vi "Send Initialize Range Controller.vi"(6 "Main Controls":refnum<vi>, 7 "Priority":T3=enum."Normal" caption="Message Priority (Normal)", 8 "error in (no error)":errorcluster, 9 "Ranges Refnum":T1, 10 "Settings":T2, 11 "Message Enqueuer in":refnum<class "Message Enqueuer.lvclass">) -> (0 "error out":errorcluster, 3 "Message Enqueuer out":refnum<class "Message Enqueuer.lvclass">)   [LabVIEW 2018, in "Range Controller.lvlib" / "Initialize Range Controller Msg.lvclass"]
doc: "Sends the <b>Range Controller.lvlib:Initialize Range Controller Msg.lvclass</b> message.\n\nThis message will call <b>Initialize Range Controller.vi</b> on the <b>Range Controller.lvlib:Range Controller Actor.lvclass</b> actor.\n\n<b>Initialize Range Controller.vi Description</b>"
uses:
  Initialize Range Controller Msg.lvclass
  <vilib>/ActorFramework/Message Enqueuer/Message Enqueuer.lvclass
  <vilib>/ActorFramework/Message Enqueuer/Message Priority.ctl
  MWWL Verification/Type Defs/ConfigSettings.ctl
  MWWL Verification/MWWL Verification/Ranges Refnum.ctl
  C:/Program Files (x86)/National Instruments/LabVIEW 2018/vi.lib/ActorFramework/Message/Message.lvclass
  Initialize Range Controller Msg.lvclass/Initialize Range Controller Msg.ctl
  <vilib>/ActorFramework/Message Enqueuer/Message Enqueuer.lvclass/Message Enqueuer.ctl
  <vilib>/ActorFramework/Message Priority Queue/Priority Enqueue.vi
  MWWL Verification/MWWL Verification.lvlib
panel:
  # "RANGES (m)"
  # "SM140"
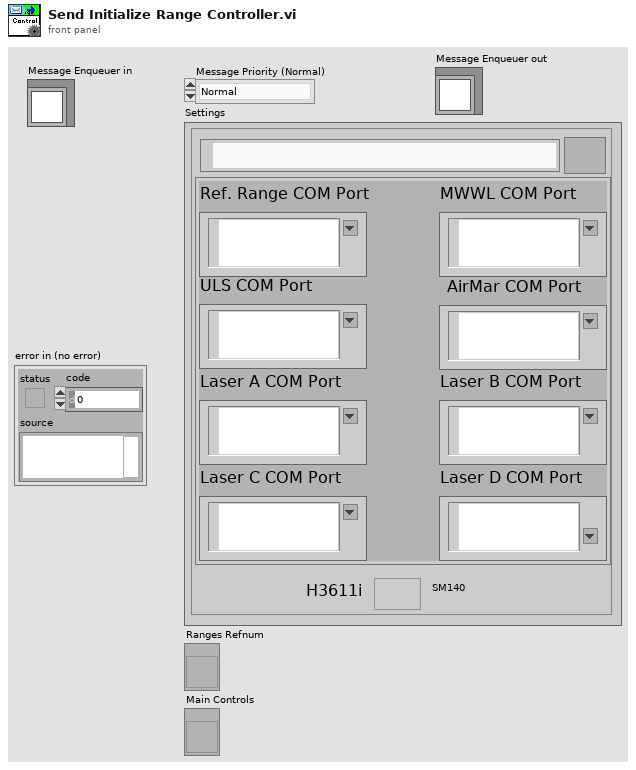
[diagram p1: front panel]
types:
  T1 = typedef "MWWL Verification.lvlib/Ranges Refnum.ctl" = refnum<vi>
  T2 = typedef "MWWL Verification.lvlib/ConfigSettings.ctl" = cluster{"Base Path":path, "DNL_Configuration Settings.Ports":cluster{"Ref. Range COM Port":refnum<visa-resource-name>, "MWWL COM Port":refnum<visa-resource-name>, "ULS COM Port":refnum<visa-resource-name>, "Laser A COM Port":refnum<visa-resource-name>, "Laser B COM Port":refnum<visa-resource-name>, "Laser C COM Port":refnum<visa-resource-name>, "Laser D COM Port":refnum<visa-resource-name>, "AirMar COM Port":refnum<visa-resource-name>}, "H3611i":bool}
  T3 = typedef "Actor Framework.lvlib/Message Enqueuer.lvclass/Message Priority.ctl" = enum16{"Low", "Normal", "High"}
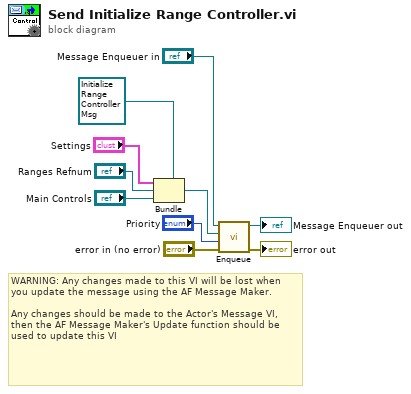
[diagram p0: block diagram]
diagram:
  # "WARNING: Any changes made to this VI will be lost when you update the message using the AF Message Maker.\n\nAny changes should be made to the Actor's Message VI, then the AF Message Maker's Update function should be used to update this VI"
  n1 = Bundle(cluster=refnum<class "Initialize Range Controller Msg.lvclass"> refnum ("Range Controller.lvlib:Initialize Range Controller Msg.lvclass"), "Settings", "Ranges Refnum", "Main Controls") -> (w6:refnum<class "Initialize Range Controller Msg.lvclass">)
  n2 = call <vilib>:"Enqueue.vi"("error in (no error)"="error in (no error)", "Message Priority (Normal)"="Priority", "Message"=w6, "Message Enqueuer in"="Message Enqueuer in") -> ("error out"=→"error out":errorcluster, "Message Enqueuer out"=→"Message Enqueuer out":refnum<class "Message Enqueuer.lvclass">)  [unwired: 6 in]
